vi "Loader.vi"(8 "error in (no error)":errorcluster, 10 "Path":path) -> (0 "error out":errorcluster)   [LabVIEW 2012, in "ServiceManagerLoader.lvclass"]
uses:
  ServiceManagerLoader.lvclass
  <vilib>/Distrio/Murmex/InitialiseMessage/InitialiseMessage.lvclass
  <vilib>/Distrio/Murmex/TerminateMessage/TerminateMessage.lvclass
  <vilib>/Distrio/Murmex/GenericMessage/GenericMessage.lvclass
  <vilib>/Distrio/Murmex/Murmex/Murmex.lvclass
  <vilib>/Distrio/Murmex/Message/Message.lvclass
panel:
  out "path":string
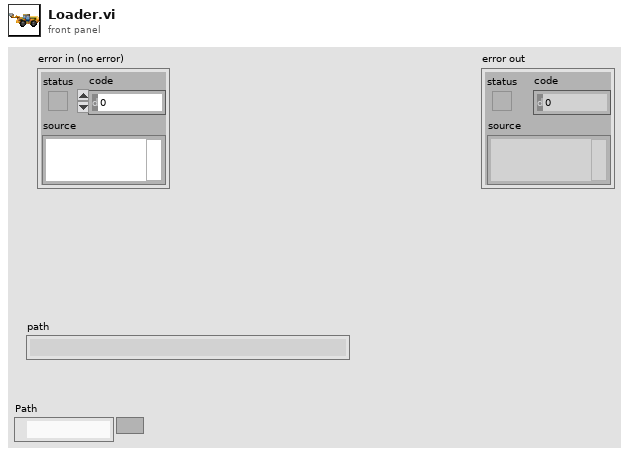
[diagram p1: front panel]
types:
  T1 = enum32{"Invalid", "Standard", "Closed", "Hidden", "Minimized", "Maximized"}
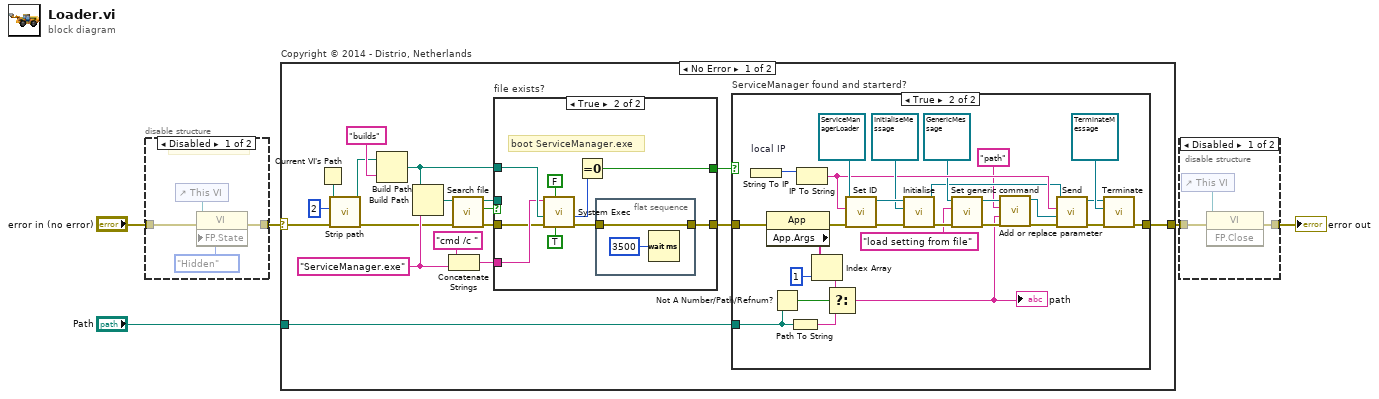
[diagram p0: block diagram]
diagram:
  n1 = disable-structure shown="Disabled" {
    disable-tunnel: "error in (no error)" -> [w7 w10]
    disable-tunnel: [w6 w10] -> w4
    frame Disabled {
      # "run minimized"
      n2 = control-ref of="This VI"() -> (w9:refnum<vi>)
      n3 = property class="VI"(reference=w9, error in=w7, "FP.State"=T1."Hidden" ("Front Panel Window:State")) -> (error out=w6:errorcluster)  [unwired: 1 out]
    }
    frame Enabled {
    }
  }
  n4 = case "Copyright © 2014 - Distrio, Netherlands" shown="No Error" w4 {
    selector: w4 -> [w15 w70]
    tunnel: [w28 w70] -> w2
    tunnel: "Path" -> [w11 _]
    frame No Error {
      w26 = "ServiceManager.exe" ("name or relative path")
      n5 = Current VI's Path() -> (path=w16:path)
      n6 = call <vilib>:"Strip path.vi"("error in (no error)"=w15, "number of strips"=2, "path in"=w16) -> ("error out"=w12:errorcluster, "path out"=w18:path)  [unwired: 7 in]
      n7 = Build Path(base path=w18, name or relative path="builds") -> (appended path=w24:path)
      n8 = Build Path(base path=w24, name or relative path=w26) -> (appended path=w23:path)
      n9 = Concatenate Strings("cmd /c " ("string"), w26) -> (w27:string)
      n10 = call <vilib>:"Search file.vi"("error in (no error)"=w12, "path in"=w23) -> ("error out"=w21:errorcluster, "found?"=w20:bool, "path out"=w22:path)  [unwired: 7 in]
      n11 = case "file exists?" shown="True" w20 {
        tunnel: w21 -> [w58 w59]
        tunnel: w22 -> [_ _]
        tunnel: w24 -> [_ w67]
        tunnel: w27 -> [_ w60]
        tunnel: [_ w63] -> w13
        tunnel: [w58 w61] -> w14
        frame False {
        }
        frame True {
          # "boot ServiceManager.exe"
          n12 = call <vilib>:"System Exec.vi"("run minimized? (F)"=TRUE, "wait until completion? (T)"=FALSE, "error in (no error)"=w59, "working directory"=w67, "command line"=w60) -> ("error out"=w62:errorcluster, "return code"=w64:i32)  [unwired: 3 in, 2 out]
          n13 = Equal To 0?(x=w64) -> (x = 0?=w63:bool)
          n14 = flat-sequence {
            tunnel: w62 -> [w68]
            tunnel: [w68] -> w61
            frame #0 {
              n15 = Wait (ms)(milliseconds to wait=u32 3500) -> ()  [unwired: 1 out]
            }
          }
        }
      }
      n16 = case "ServiceManager found and starterd?" shown="True" w13 {
        tunnel: [w29 w55] -> w28
        tunnel: w14 -> [w29 w50]
        tunnel: w11 -> [_ w47]
        frame False {
        }
        frame True {
          n17 = String To IP "local IP"() -> (0:w56:u32)  [unwired: 1 in]
          n18 = property class="App"(error in=w50) -> (error out=w52:errorcluster, "App.Args"=w51:string[])  [unwired: 1 in, 1 out]
          n19 = Not A Number/Path/Refnum?(number/path/refnum=w47) -> (NaN/Path/Refnum?=w48:bool)
          n20 = Path To String(path=w47) -> (string=w46:string)
          n21 = IP To String(2:w56) -> (0:w40:string)  [unwired: 1 in]
          n22 = Index Array(array=w51, index=1) -> (element=w45:string)
          n23 = Select(t=w45, s=w48, f=w46) -> (s? t:f=w30:string)
          "path" <- w30
          n24 = call <vilib>:"Set ID.vi"("error in (no error)"=w52, "id"=w40, "Murmex in"=refnum<class "ServiceManagerLoader.lvclass"> refnum ("ServiceManagerStarter in")) -> ("error out"=w53:errorcluster, "Murmex out"=w54:refnum<class "ServiceManagerLoader.lvclass">)  [unwired: 7 in]
          n25 = call-dynamic "Initialise.vi"("error in (no error)"=w53, "Message in"=refnum<class "InitialiseMessage.lvclass"> refnum, "Murmex in"=w54) -> ("error out"=w37:errorcluster, "Murmex out"=w32:refnum<class "ServiceManagerLoader.lvclass">)  [unwired: 7 in]
          n26 = call <vilib>:"Set generic command.vi"("error in (no error)"=w37, "generic command"="load setting from file" ("command string"), "GenericMessage in"=refnum<class "GenericMessage.lvclass"> refnum ("Distrio Murmex 1.5:GenericMessage")) -> ("error out"=w36:errorcluster, "GenericMessage out"=w38:refnum<class "GenericMessage.lvclass">)  [unwired: 7 in]
          n27 = call <vilib>:"Add or replace parameter.vi"("error in (no error)"=w36, "value"=w30, "name"="path", "Message in"=w38) -> ("error out"=w35:errorcluster, "Message out"=w33:refnum<class "GenericMessage.lvclass">)  [unwired: 6 in]
          n28 = call <vilib>:"Send.vi"("error in (no error)"=w35, "Message"=w33, "recipient"=w40, "Murmex in"=w32) -> ("error out"=w42:errorcluster, "Murmex out"=w41:refnum<class "ServiceManagerLoader.lvclass">)  [unwired: 6 in]
          n29 = call-dynamic "Terminate.vi"("error in (no error)"=w42, "Message in"=refnum<class "TerminateMessage.lvclass"> refnum, "Murmex in"=w41) -> ("error out"=w55:errorcluster)  [unwired: 7 in, 1 out]
        }
      }
    }
    frame Error {
    }
  }
  n30 = disable-structure shown="Disabled" {
    disable-tunnel: [w72 w74] -> w3
    disable-tunnel: w2 -> [w71 w74]
    frame Disabled {
      n31 = control-ref of="This VI"() -> (w73:refnum<vi>)
      n32 = invoke class="VI" method="FP.Close"(reference=w73, error in=w71) -> (error out=w72:errorcluster)  [unwired: 1 in, 2 out]
    }
    frame Enabled {
    }
  }
  "error out" <- w3
